vi "Untitled 1.vi"(11 "Data In":T3={"Time Limit"=1000, "Length"=0, "Memory"=[], "Barrier"=[[-1, -1, -1], [-1, -255, -1], [-1, -1, -1]], "Snake"=[[-1, -1, -1], [-1, -255, -1], [-1, -1, -1]], "Tail"=[[-1, -1, -1], [-1, -255, -1], [-1, -1, -1]], "Food"=[[-1, -1, -1], [-1, -255, -1], [-1, -1, -1]]}) -> (3 "Data Out":T1)   [LabVIEW 2020]
uses:
  Snake TypeDef/Snake DataIn TypeDef.ctl
  Snake TypeDef/Snake DataOut TypeDef.ctl
  TypeDef/Direction_TypeDef.ctl
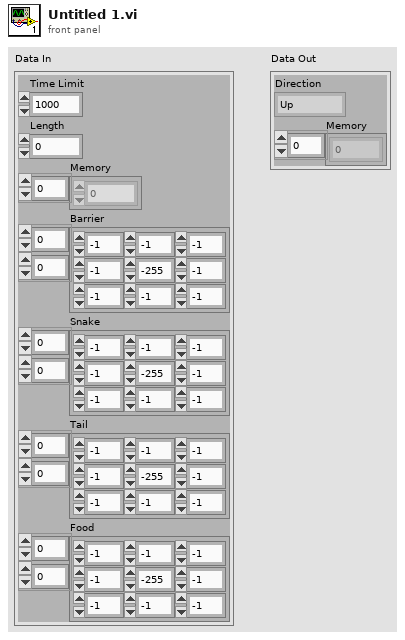
[diagram p1: front panel]
types:
  T1 = typedef "Snake DataOut TypeDef.ctl" = cluster{"Direction":T2, "Memory":u8[]}
  T2 = typedef "Direction_TypeDef.ctl" = enum8{"Up", "Down", "Left", "Right"}
  T3 = typedef "Snake DataIn TypeDef.ctl" = cluster{"Time Limit":i32, "Length":i32, "Memory":u8[], "Barrier":i32[][], "Snake":i32[][], "Tail":i32[][], "Food":i32[][]}
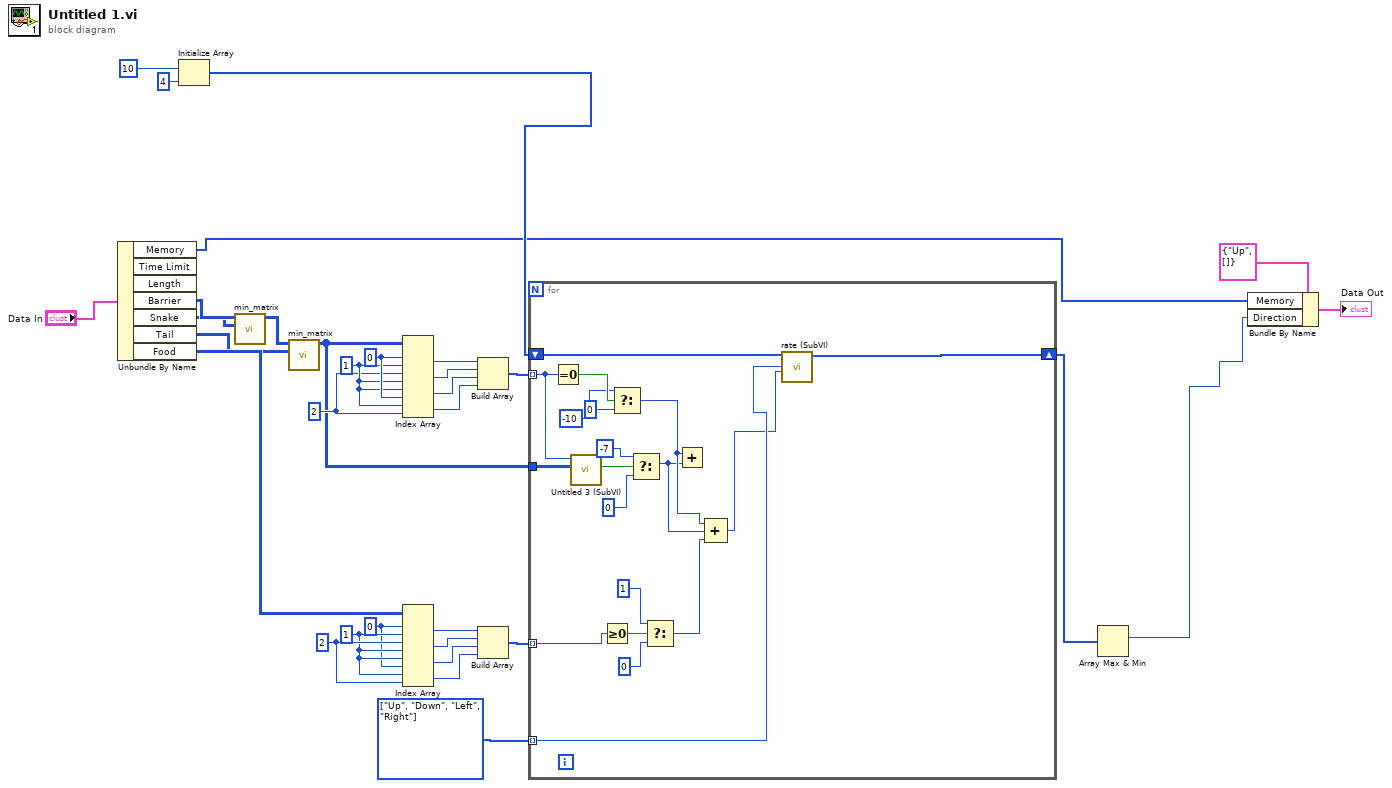
[diagram p0: block diagram]
diagram:
  w18 = 2 ("index (row)")
  w17 = 1 ("disabled index (col)")
  w16 = 0 ("index (row)")
  w27 = 2 ("index (row)")
  w12 = T2[] [enum."Up", enum."Down", enum."Left", enum."Right"] items=["Up", "Down", "Left", "Right"] ("Array")
  w28 = 1 ("disabled index (col)")
  w29 = 0 ("index (row)")
  n1 = Unbundle By Name("Data In") -> ("Memory"=w1:u8[], "Barrier"=w11:i32[][], "Snake"=w10:i32[][], "Tail"=w8:i32[][], "Food"=w15:i32[][])  [unwired: 2 out]
  n2 = Initialize Array(10 ("dimension size"), 4 ("dimension size")) -> (w5:i32[])
  n3 = call "min_matrix.vi"("Array 3"=w10, "Array in"=w11) -> ("Array out"=w9:i32[][])  [unwired: 9 in]
  n4 = call "min_matrix.vi"("Array 3"=w8, "Array in"=w9) -> ("Array out"=w4:i32[][])  [unwired: 9 in]
  n5 = Index Array(array=w4, index (row) #1=w29, index (col) #1=w28, index (row) #2=w27, index (col) #2=w28, index (row) #3=w28, index (col) #3=w29, index (row) #4=w28, index (col) #4=w27) -> (element #1=w26:i32, element #2=w25:i32, element #3=w24:i32, element #4=w23:i32)
  n6 = Index Array(array=w15, index (row) #1=w16, index (col) #1=w17, index (row) #2=w18, index (col) #2=w17, index (row) #3=w17, index (col) #3=w16, index (row) #4=w17, index (col) #4=w18) -> (element #1=w19:i32, element #2=w20:i32, element #3=w21:i32, element #4=w22:i32)
  n7 = Build Array(w26, w25, w24, w23) -> (w14:i32[])
  n8 = Build Array(w19, w20, w21, w22) -> (w13:i32[])
  n9 = for {
    tunnel: w14 -> [w47] mode=indexing
    tunnel: w13 -> [w38] mode=indexing
    tunnel: w12 -> [w51] mode=indexing
    shift-right: [w49] -> w3
    shift-left: w5 -> [w50]
    tunnel: w4 -> [w48]
    n10 = Equal To 0?(x=w47) -> (x = 0?=w46:bool)
    n11 = call "Untitled 3 (SubVI).vi"("Array in"=w48, "Memory in"=w47) -> ("Boolean"=w43:bool)  [unwired: 8 in, 1 out]
    n12 = Greater Or Equal To 0?(x=w38) -> (x >= 0?=w37:bool)
    n13 = Select(t=-10 ("dimension size"), s=w46, f=0) -> (s? t:f=w40:i32)
    n14 = Select(t=-7 ("dimension size"), s=w43, f=0) -> (s? t:f=w39:i32)
    n15 = Select(t=1 ("f"), s=w37, f=0) -> (s? t:f=w34:i32)
    n16 = Add(x=w40, y=w39) -> ()  [unwired: 1 out]
    n17 = Compound Arithmetic op=ADD(w40, w39, w34) -> (w33:i32)
    n18 = call "rate (SubVI).vi"("new element/subarray"=w33, "direction"=w51, "Array in"=w50) -> ("Array out"=w49:i32[])  [unwired: 8 in]
  }
  n19 = Array Max & Min(array=w3) -> (max index (indices)=w2:i32)  [unwired: 3 out]
  n20 = Bundle By Name(cluster=T1 {"Direction"=enum."Up", "Memory"=[]} ("Data Out"), "Memory"=w1, "Direction"=w2) -> (→"Data Out":T1)
